vi "ExamineRowOfTrees.vi"(6 "ReversSearchDirection":bool, 8 "Row/Column":i32, 9 "Column":bool, 10 "MapIn":u8[][](array[numeric]), 11 "TreesVisiableIn":set{cluster{"Row":i32, "Column":i32}}(c389)) -> (3 "TreesVisiableOut":set{cluster{"Row":i32, "Column":i32}}(c389))   [LabVIEW 2020, in "2022_8.lvclass"]
uses:
  2022_8.lvclass
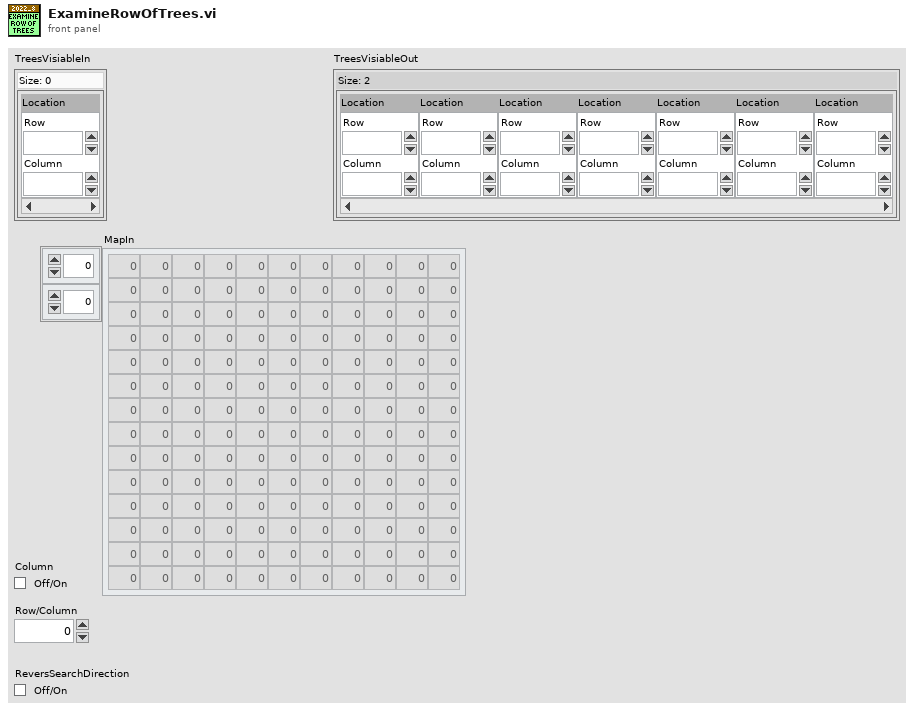
[diagram p1: front panel]
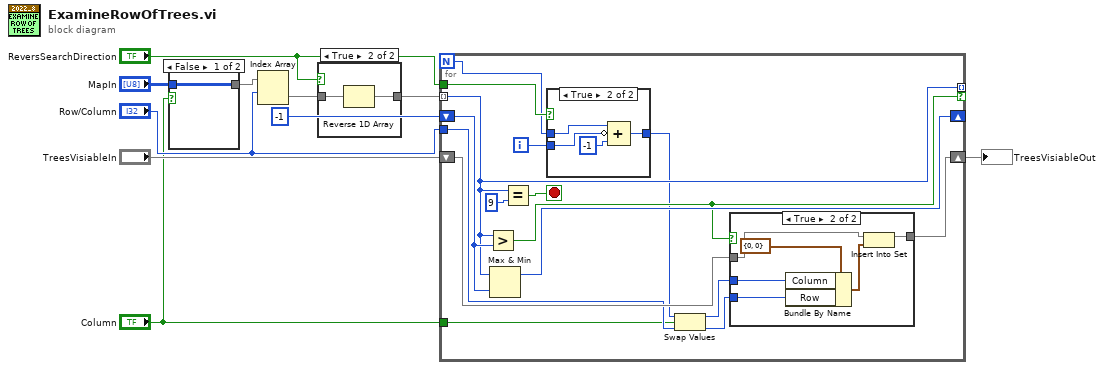
[diagram p0: block diagram]
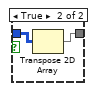
[diagram p3: hidden frame]
diagram:
  n1 = case shown="False" "Column" {
    tunnel: "MapIn" -> [w11 w13]
    tunnel: [w11 w12] -> w8
    frame False {
    }
    frame True {
      n2 = Transpose 2D Array(2D array=w13) -> (transposed array=w12:u8[][])
    }
  }
  n3 = Index Array(array=w8, index (row)="Row/Column") -> (element=w3:u8[])  [unwired: 1 in]
  n4 = case shown="True" "ReversSearchDirection" {
    tunnel: w3 -> [w14 w16]
    tunnel: [w14 w15] -> w2
    frame False {
    }
    frame True {
      n5 = Reverse 1D Array(array=w16) -> (reversed array=w15:u8[])
    }
  }
  n6 = for {
    N -> [w17]
    tunnel: w2 -> [w28] mode=indexing
    shift-right: [w29] -> _
    shift-left: -1 -> [w30]
    tunnel: [w28] -> _ mode=indexing if=w27
    shift-right: [w25] -> w6
    shift-left: "TreesVisiableIn" -> [w26]
    tunnel: "Row/Column" -> [w24]
    tunnel: "Column" -> [w23]
    tunnel: "ReversSearchDirection" -> [w20]
    i -> [w19]
    stop <- w31 stop-if-true
    n7 = Greater?(x=w28, y=w30) -> (0:w27:bool)
    n8 = Max & Min(x=w28, y=w30) -> (max(x,y)=w29:i32)  [unwired: 1 out]
    n9 = Equal?(x=w28, y=u8 9) -> (x = y?=w31:bool)
    n10 = case shown="True" w20 {
      tunnel: w19 -> [w33 w34]
      tunnel: [w33 w35] -> w18
      tunnel: w17 -> [_ w37]
      frame False {
      }
      frame True {
        n11 = Compound Arithmetic op=ADD(w37, invert w34, -1 ("value")) -> (w35:i32)
      }
    }
    n12 = Swap Values(12:w18, 13:w23, 14:w24) -> (1:w22:i32, 3:w21:i32)
    n13 = case shown="True" w27 {
      tunnel: w26 -> [w38 w44]
      tunnel: [w38 w43] -> w25
      tunnel: w22 -> [_ w40]
      tunnel: w21 -> [_ w39]
      frame False {
      }
      frame True {
        n14 = Bundle By Name(cluster=cluster{"Row":i32, "Column":i32} {"Row"=0, "Column"=0} ("element"), "Column"=w40, "Row"=w39) -> (w41:cluster{"Row":i32, "Column":i32})
        n15 = Insert Into Set(10:w41, 11:w44) -> (3:w43:set{cluster{"Row":i32, "Column":i32}})  [unwired: 1 out]
      }
    }
  }
  "TreesVisiableOut" <- w6
